vi "Cluster Shifter by 2.vi"(8 "Input Valid":bool, 10 "Acquisition Status In":T1={"Reset"=FALSE, "Acquisition Engine Start (Arm)"=FALSE, "Current State"=enum."Acquire Pre-Trigger Samples", "Trig Offset"=0, "Points Unread"=0, "Points Acquired"=0, "Records Done"=0, "Start of Read"=FALSE, "End of Read"=FALSE, "Start of Record"=FALSE, "End of Record"=FALSE, "Ready for Ref Trig"=FALSE, "In Reset?"=FALSE}, 11 "Current Data":T3) -> (0 "Output Data Valid":bool, 2 "Acquisition StatusOut":T1={"Reset"=FALSE, "Acquisition Engine Start (Arm)"=FALSE, "Current State"=enum."Acquire Pre-Trigger Samples", "Trig Offset"=0, "Points Unread"=0, "Points Acquired"=0, "Records Done"=0, "Start of Read"=FALSE, "End of Read"=FALSE, "Start of Record"=FALSE, "End of Record"=FALSE, "Ready for Ref Trig"=FALSE, "In Reset?"=FALSE}, 3 "Shifted Data":T3)   [LabVIEW 2012]
doc: "This VI shifts input data based on shift input. The maximum shift of this VI is one sample clock tick.\nThis VI combines data from two consecutive samples based on shifter position. This is useful when combining data from parallel streams based on trigger position.\n\n\n<b> Latency = 0 Ticks </b>"
uses:
  <userlib>/OCT Reference Design/Acquisition Engine/Multi-Channel Analog Input Data.ctl
  <userlib>/OCT Reference Design/Acquisition Engine/Acquisition Status.ctl
  <userlib>/OCT Reference Design/Acquisition Engine/Acquisition Engine State.ctl
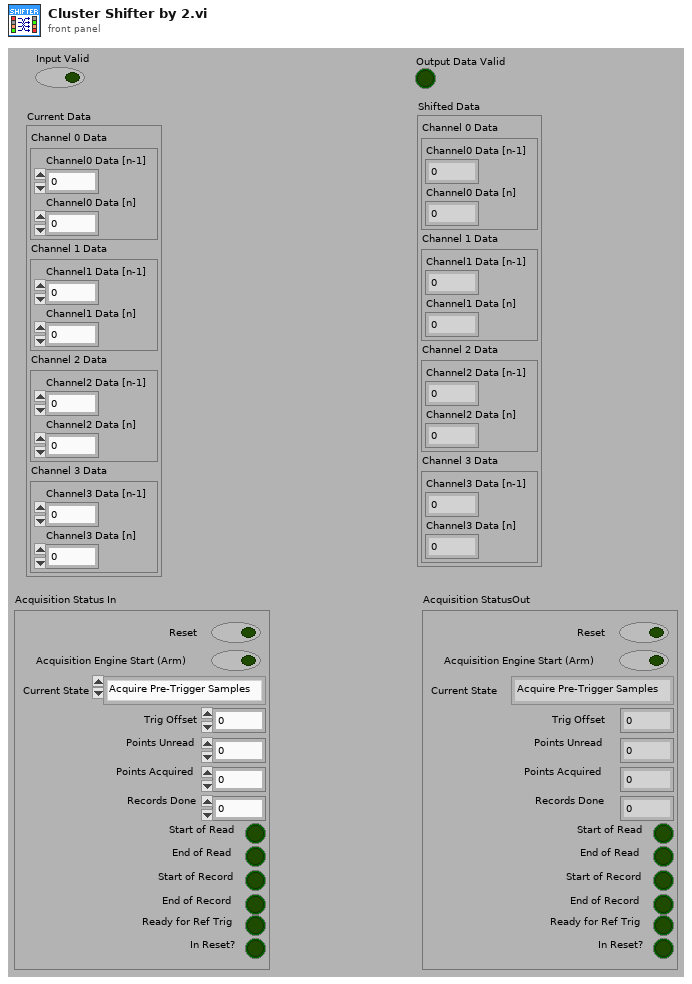
[diagram p1: front panel]
types:
  T1 = typedef "Acquisition Status.ctl" = cluster{"Reset":bool, "Acquisition Engine Start (Arm)":bool, "Current State":T2, "Trig Offset":u8, "Points Unread":u16, "Points Acquired":u16, "Records Done":u16, "Start of Read":bool, "End of Read":bool, "Start of Record":bool, "End of Record":bool, "Ready for Ref Trig":bool, "In Reset?":bool}
  T2 = typedef "Acquisition Engine State.ctl" = enum8{"Idle", "Arm Acquisition Engine", "Acquire Pre-Trigger Samples", "Wait for Trigger", "Acquisition Hold Off Time", "Read Data from Buffer", "Check Records Done?", "Re-Arm State", "Flush Available Data"}
  T3 = typedef "Multi-Channel Analog Input Data.ctl" = cluster{"Channel 0 Data":cluster{"Channel0 Data [n-1]":i16, "Channel0 Data [n]":i16}, "Channel 1 Data":cluster{"Channel1 Data [n-1]":i16, "Channel1 Data [n]":i16}, "Channel 2 Data ":cluster{"Channel2 Data [n-1]":i16, "Channel2 Data [n]":i16}, "Channel 3 Data":cluster{"Channel3 Data [n-1]":i16, "Channel3 Data [n]":i16}}
  T4 = cluster{"Channel 0 Data":cluster{"Channel0 Data [n-1]":i16, "Channel0 Data [n]":i16}, "Channel 1 Data":cluster{"Channel1 Data [n-1]":i16, "Channel1 Data [n]":i16}, "Channel 2 Data ":cluster{"Channel2 Data [n-1]":i16, "Channel2 Data [n]":i16}, "Channel 3 Data":cluster{"Channel3 Data [n-1]":i16, "Channel3 Data [n]":i16}}
  T5 = cluster{"Previous Data":cluster{"Channel 0 Data":cluster{"Channel0 Data [n-1]":i16, "Channel0 Data [n]":i16}, "Channel 1 Data":cluster{"Channel1 Data [n-1]":i16, "Channel1 Data [n]":i16}, "Channel 2 Data ":cluster{"Channel2 Data [n-1]":i16, "Channel2 Data [n]":i16}, "Channel 3 Data":cluster{"Channel3 Data [n-1]":i16, "Channel3 Data [n]":i16}}, "Previous Data Valid":bool}
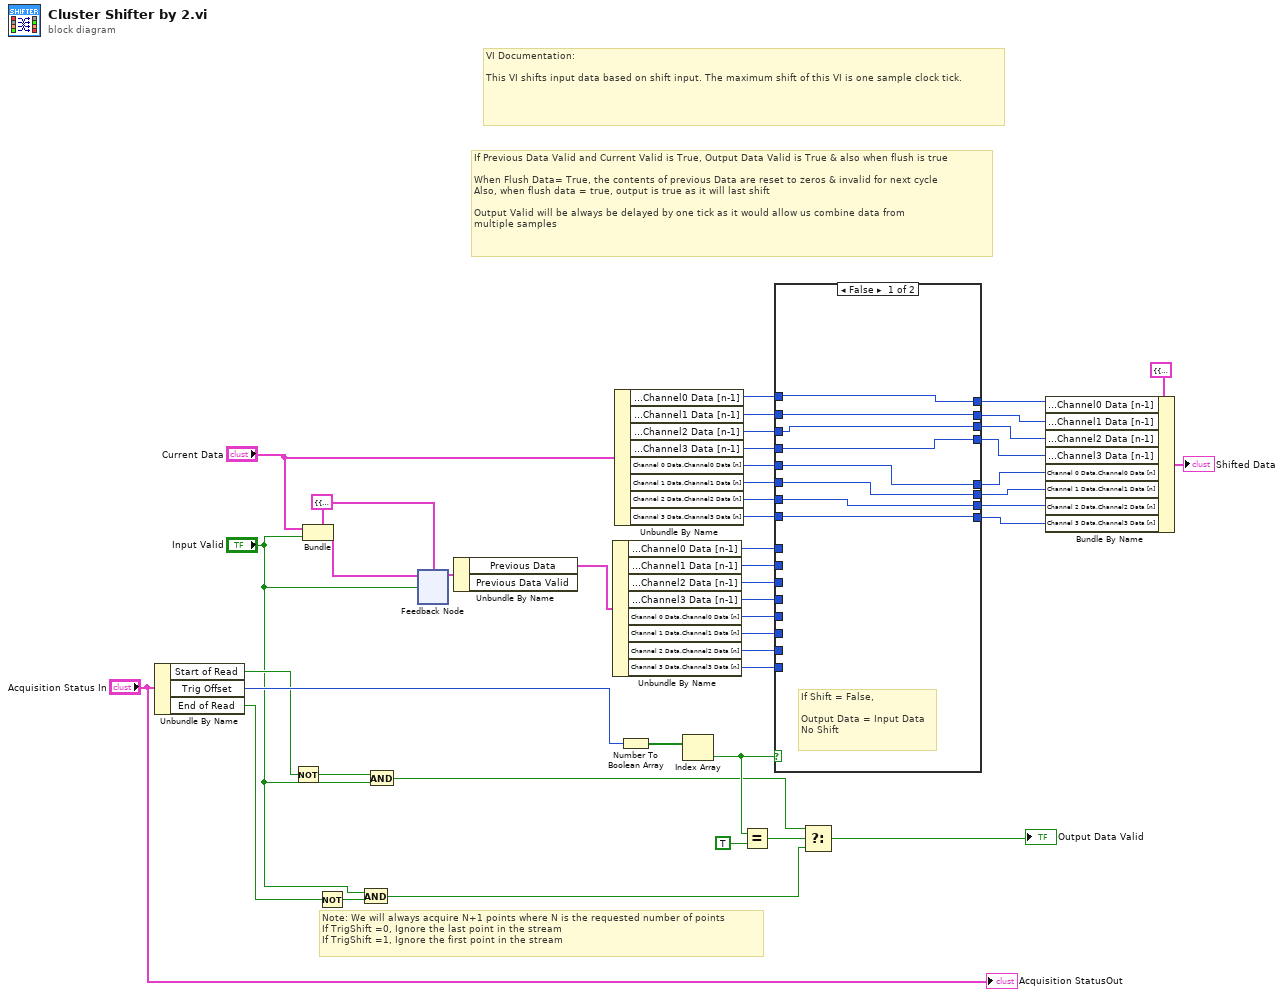
[diagram p0: block diagram]
diagram:
  w42 = T5 {"Previous Data"={"Channel 0 Data"={"Channel0 Data [n-1]"=0, "Channel0 Data [n]"=0}, "Channel 1 Data"={"Channel1 Data [n-1]"=0, "Channel1 Data [n]"=0}, "Channel 2 Data "={"Channel2 Data [n-1]"=0, "Channel2 Data [n]"=0}, "Channel 3 Data"={"Channel3 Data [n-1]"=0, "Channel3 Data [n]"=0}}, "Previous Data Valid"=FALSE} ("cluster")
  # "Note: We will always acquire N+1 points where N is the requested number of points\nIf TrigShift =0, Ignore the last point in the stream\nIf TrigShift =1, Ignore the first point in the stream"
  # "VI Documentation:\n\nThis VI shifts input data based on shift input. The maximum shift of this VI is one sample clock tick."
  # "If Previous Data Valid and Current Valid is True, Output Data Valid is True & also when flush is true\n\nWhen Flush Data= True, the contents of previous Data are reset to zeros & invalid for next cycle\nAlso, when flush data = true, output is true as it will last shift\n\nOutput Valid will be always be delayed by one tick as it would allow us combine data from\nmultiple samples"
  n1 = Unbundle By Name("Acquisition Status In") -> ("Start of Read"=w5:bool, "Trig Offset"=w7:u8, "End of Read"=w6:bool)
  n2 = Not(x=w5) -> (.not. x?=w2:bool)
  n3 = Bundle(cluster=w42, "Previous Data"="Current Data", "Previous Data Valid"="Input Valid") -> (w43:T5)
  n4 = Not(x=w6) -> (.not. x?=w10:bool)
  n5 = And(x="Input Valid", y=w10) -> (x .and. y?=w9:bool)
  n6 = And(x=w2, y="Input Valid") -> (x .and. y?=w3:bool)
  n7 = feedback-in #1(w43, "Input Valid") -> ()
  n8 = feedback #1(w42) -> (w44:T5)
  n9 = Unbundle By Name(w44) -> ("Previous Data"=w33:T4)  [unwired: 1 out]
  n10 = Unbundle By Name(w33) -> ("Channel 0 Data.Channel0 Data [n-1]"=w32:i16, "Channel 1 Data.Channel1 Data [n-1]"=w31:i16, "Channel 2 Data.Channel2 Data [n-1]"=w30:i16, "Channel 3 Data.Channel3 Data [n-1]"=w29:i16, "Channel 0 Data.Channel0 Data [n]"=w28:i16, "Channel 1 Data.Channel1 Data [n]"=w27:i16, "Channel 2 Data.Channel2 Data [n]"=w26:i16, "Channel 3 Data.Channel3 Data [n]"=w25:i16)
  n11 = Unbundle By Name("Current Data") -> ("Channel 0 Data.Channel0 Data [n-1]"=w41:i16, "Channel 1 Data.Channel1 Data [n-1]"=w40:i16, "Channel 2 Data.Channel2 Data [n-1]"=w39:i16, "Channel 3 Data.Channel3 Data [n-1]"=w38:i16, "Channel 0 Data.Channel0 Data [n]"=w37:i16, "Channel 1 Data.Channel1 Data [n]"=w36:i16, "Channel 2 Data.Channel2 Data [n]"=w35:i16, "Channel 3 Data.Channel3 Data [n]"=w34:i16)
  n12 = Number To Boolean Array(number=w7) -> (Boolean array=w45:bool[])
  n13 = Index Array(array=w45) -> (element=w14:bool)  [unwired: 1 in]
  n14 = Equal?(x=w14, y=TRUE) -> (x = y?=w12:bool)
  n15 = case shown="False" w14 {
    tunnel: w41 -> [w53 w57]
    tunnel: w40 -> [w52 w56]
    tunnel: w39 -> [w51 w55]
    tunnel: w38 -> [w50 w54]
    tunnel: w37 -> [w49 _]
    tunnel: w36 -> [w48 _]
    tunnel: w35 -> [w47 _]
    tunnel: w34 -> [w46 _]
    tunnel: w32 -> [_ _]
    tunnel: w31 -> [_ _]
    tunnel: w30 -> [_ _]
    tunnel: w29 -> [_ _]
    tunnel: w28 -> [_ w61]
    tunnel: w27 -> [_ w60]
    tunnel: w26 -> [_ w59]
    tunnel: w25 -> [_ w58]
    tunnel: [w53 w61] -> w24
    tunnel: [w52 w60] -> w23
    tunnel: [w51 w59] -> w22
    tunnel: [w50 w58] -> w21
    tunnel: [w49 w57] -> w20
    tunnel: [w48 w56] -> w19
    tunnel: [w47 w55] -> w18
    tunnel: [w46 w54] -> w17
    frame False {
      # "If Shift = False,\n\nOutput Data = Input Data\nNo Shift"
    }
    frame True {
      # "Previous Input N => Current N-1\nCurrent  Input N  => Current N"
    }
  }
  n16 = Select(t=w3, s=w12, f=w9) -> (s? t:f=→"Output Data Valid":bool)
  n17 = Bundle By Name(cluster=T4 {"Channel 0 Data"={"Channel0 Data [n-1]"=0, "Channel0 Data [n]"=0}, "Channel 1 Data"={"Channel1 Data [n-1]"=0, "Channel1 Data [n]"=0}, "Channel 2 Data "={"Channel2 Data [n-1]"=0, "Channel2 Data [n]"=0}, "Channel 3 Data"={"Channel3 Data [n-1]"=0, "Channel3 Data [n]"=0}} ("Current Data"), "Channel 0 Data.Channel0 Data [n-1]"=w24, "Channel 1 Data.Channel1 Data [n-1]"=w23, "Channel 2 Data.Channel2 Data [n-1]"=w22, "Channel 3 Data.Channel3 Data [n-1]"=w21, "Channel 0 Data.Channel0 Data [n]"=w20, "Channel 1 Data.Channel1 Data [n]"=w19, "Channel 2 Data.Channel2 Data [n]"=w18, "Channel 3 Data.Channel3 Data [n]"=w17) -> (→"Shifted Data":T4)
  "Acquisition StatusOut" <- "Acquisition Status In"
